vi "_fast_cmd_compose.vi"(0 "Double in (0.0)":dbl, 4 "Int32 in (0)":i32, 5 "*WAI (F)":bool, 6 "Int64 in (0)":i64, 7 "Data Type in":i32, 8 "Boolean in (F)":bool, 9 "String in (\"\")":string, 10 "Direct cmd in":string, 11 "SCPI Command without parameter":string) -> (2 "Direct cmd out":string, 3 "Complete SCPI Command":string)   [LabVIEW 2020, in "Rohde&Schwarz RTx Oscilloscopes.lvlib" / "rsidr_core.lvlib"]
uses:
  rsidr_core.lvlib
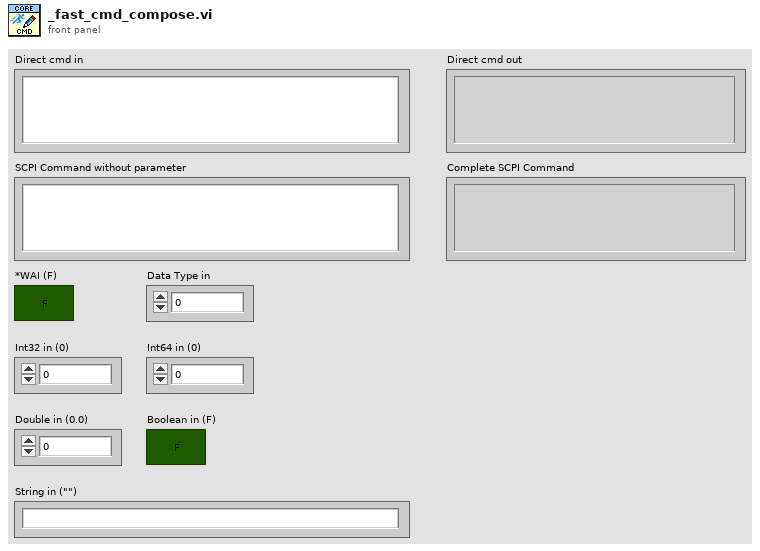
[diagram p1: front panel]
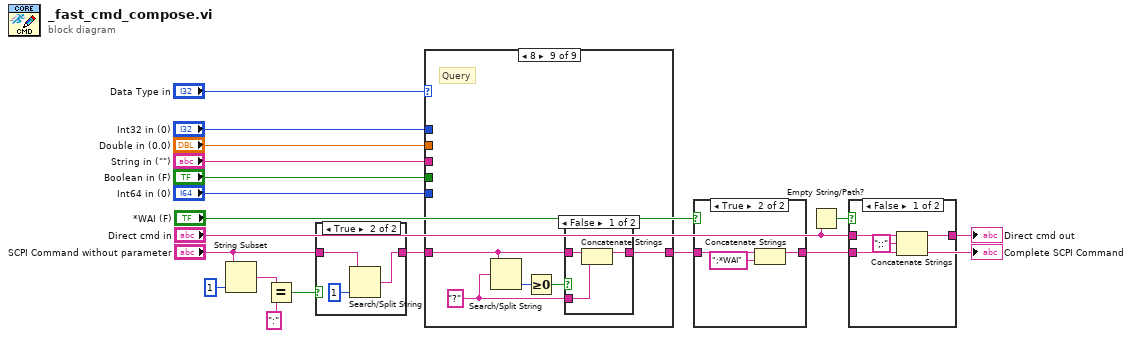
[diagram p0: block diagram]
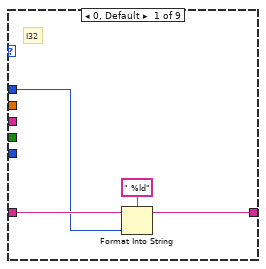
[diagram p5: hidden frame]
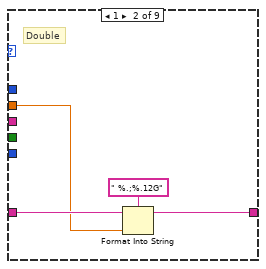
[diagram p6: hidden frame]
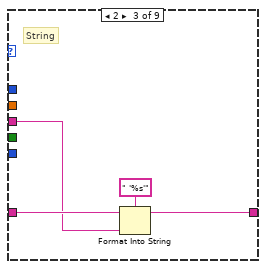
[diagram p7: hidden frame]
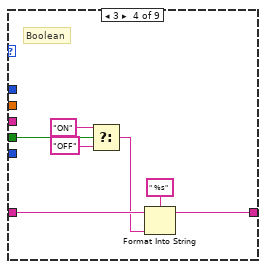
[diagram p8: hidden frame]
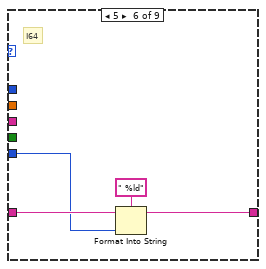
[diagram p10: hidden frame]
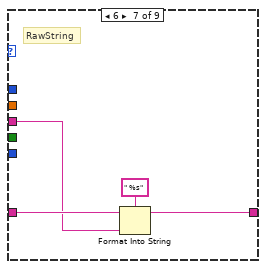
[diagram p11: hidden frame]
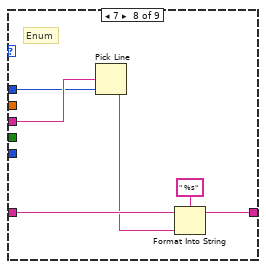
[diagram p12: hidden frame]
diagram:
  n1 = String Subset(string="SCPI Command without parameter", length (rest)=1 ("length (rest)")) -> (substring=w6:string)  [unwired: 1 in]
  n2 = Equal?(x=w6, y=":" ("search string/char (-)")) -> (x = y?=w4:bool)
  n3 = case shown="True" w4 {
    tunnel: "SCPI Command without parameter" -> [w19 w22]
    tunnel: [w19 w20] -> w12
    frame False {
    }
    frame True {
      n4 = Search/Split String(string=w22, offset (0)=1) -> (match + rest of string=w20:string)  [unwired: 1 in, 2 out]
    }
  }
  n5 = case shown="8" "Data Type in" {
    tunnel: "Int32 in (0)" -> [w24 _ _ _ _ _ _ w51 _]
    tunnel: w12 -> [w25 w29 w33 w40 w42 w45 w49 w55 w59]
    tunnel: [w23 w28 w32 w39 w42 w44 w48 w54 w58] -> w2
    tunnel: "Double in (0.0)" -> [_ w27 _ _ _ _ _ _ _]
    tunnel: "String in (\"\")" -> [_ _ w31 _ _ _ w47 w53 _]
    tunnel: "Boolean in (F)" -> [_ _ _ w36 _ _ _ _ _]
    tunnel: "Int64 in (0)" -> [_ _ _ _ _ w43 _ _ _]
    frame 0, Default {
      # "I32"
      n6 = Format Into String(format string=" %ld", initial string=w25, w24) -> (resulting string=w23:string)  [unwired: 1 in, 1 out]
    }
    frame 1 {
      # "Double"
      n7 = Format Into String(format string=" %.;%.12G", initial string=w29, w27) -> (resulting string=w28:string)  [unwired: 1 in, 1 out]
    }
    frame 2 {
      # "String"
      n8 = Format Into String(format string=" '%s'", initial string=w33, w31) -> (resulting string=w32:string)  [unwired: 1 in, 1 out]
    }
    frame 3 {
      # "Boolean"
      n9 = Select(t="ON", s=w36, f="OFF") -> (s? t:f=w35:string)
      n10 = Format Into String(format string=" %s", initial string=w40, w35) -> (resulting string=w39:string)  [unwired: 1 in, 1 out]
    }
    frame 4 {
      # "Event"
    }
    frame 5 {
      # "I64"
      n11 = Format Into String(format string=" %ld", initial string=w45, w43) -> (resulting string=w44:string)  [unwired: 1 in, 1 out]
    }
    frame 6 {
      # "RawString"
      n12 = Format Into String(format string=" %s", initial string=w49, w47) -> (resulting string=w48:string)  [unwired: 1 in, 1 out]
    }
    frame 7 {
      # "Enum"
      n13 = Pick Line(multi-line string=w53, line index=w51) -> (output string=w52:string)  [unwired: 1 in]
      n14 = Format Into String(format string=" %s", initial string=w55, w52) -> (resulting string=w54:string)  [unwired: 1 in, 1 out]
    }
    frame 8 {
      w61 = "?" ("search string/char (-)")
      # "Query"
      n15 = Search/Split String(string=w59, search string/char (-)=w61) -> (offset of match=w60:i32)  [unwired: 1 in, 2 out]
      n16 = Greater Or Equal To 0?(x=w60) -> (x >= 0?=w57:bool)
      n17 = case shown="False" w57 {
        tunnel: w61 -> [w63 _]
        tunnel: w59 -> [w64 w65]
        tunnel: [w62 w65] -> w58
        frame False {
          n18 = Concatenate Strings(w64, w63) -> (w62:string)
        }
        frame True {
        }
      }
    }
  }
  n19 = case shown="True" "*WAI (F)" {
    tunnel: w2 -> [w66 w69]
    tunnel: [w66 w68] -> w1
    frame False {
    }
    frame True {
      n20 = Concatenate Strings(w69, ";*WAI" ("string")) -> (w68:string)
    }
  }
  "Complete SCPI Command" <- w1
  n21 = Empty String/Path?(string/path="Direct cmd in") -> (empty?=w11:bool)
  n22 = case shown="False" w11 {
    tunnel: w1 -> [w71 w74]
    tunnel: "Direct cmd in" -> [w73 _]
    tunnel: [w70 w74] -> w9
    frame False {
      n23 = Concatenate Strings(w73, ";:" ("string"), w71) -> (w70:string)
    }
    frame True {
    }
  }
  "Direct cmd out" <- w9
